vi "FTW-WebService-InitializeRouter.vi"(5 "Default Request Timeout":i32 format="%dmsec", 11 "error in":errorcluster) -> (4 "Incoming HTTP Request":refnum<event-registration>, 15 "error out":errorcluster)   [LabVIEW 2015, in "FTW-WebService.lvclass"]
uses:
  FTW-WebService.lvclass
panel:
  # "Inputs"
  # "Outputs"
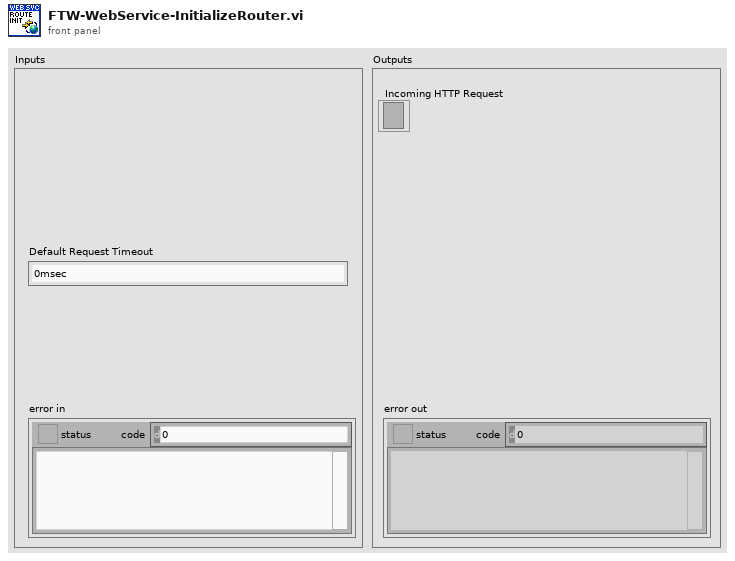
[diagram p1: front panel]
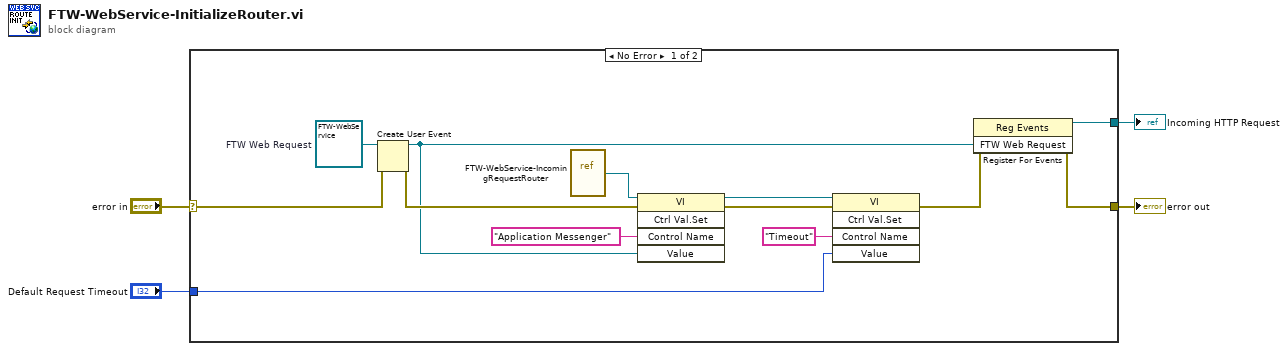
[diagram p0: block diagram]
diagram:
  n1 = case shown="No Error" "error in" {
    selector: "error in" -> [w10 w18]
    tunnel: [w7 w18] -> w4
    tunnel: "Default Request Timeout" -> [w12 _]
    tunnel: [w5 _] -> w1
    frame No Error {
      w11 = refnum<class "FTW-WebService.lvclass"> refnum  # FTW Web Request
      n2 = Create User Event(user event datatype=w11, error in=w10) -> (user event=w6:refnum<user-event>, error out=w9:errorcluster)
      n3 = vi-ref "FTW-WebService-IncomingRequestRouter.vi"() -> (w17:refnum<vi>)
      n4 = invoke class="VI" method="Ctrl Val.Set"(reference=w17, error in=w9, "Control Name"="Application Messenger", "Value"=w6) -> (reference out=w15:refnum<vi>, error out=w14:errorcluster)  [unwired: 1 in, 3 out]
      n5 = invoke class="VI" method="Ctrl Val.Set"(reference=w15, error in=w14, "Control Name"="Timeout", "Value"=w12) -> (error out=w8:errorcluster)  [unwired: 1 in, 4 out]
      n6 = register-events(error in=w8, w6) -> (reference out=w5:refnum<event-registration>, error out=w7:errorcluster)  [unwired: 1 in]
    }
    frame Error {
    }
  }
  "error out" <- w4
  "Incoming HTTP Request" <- w1
